vi "ReadMeanStdDevTrac.vi"(10 "error in":errorcluster, 11 "reference in 3":refnum<visa-resource-name>) -> (0 "error out 2":errorcluster, 1 "STDDEV":string, 2 "MEAN":string, 3 "TRACEr":string, 5 "reference out 4":refnum<visa-resource-name>)   [LabVIEW 2009]
panel:
  out "error out":errorcluster
  out "return count":u32
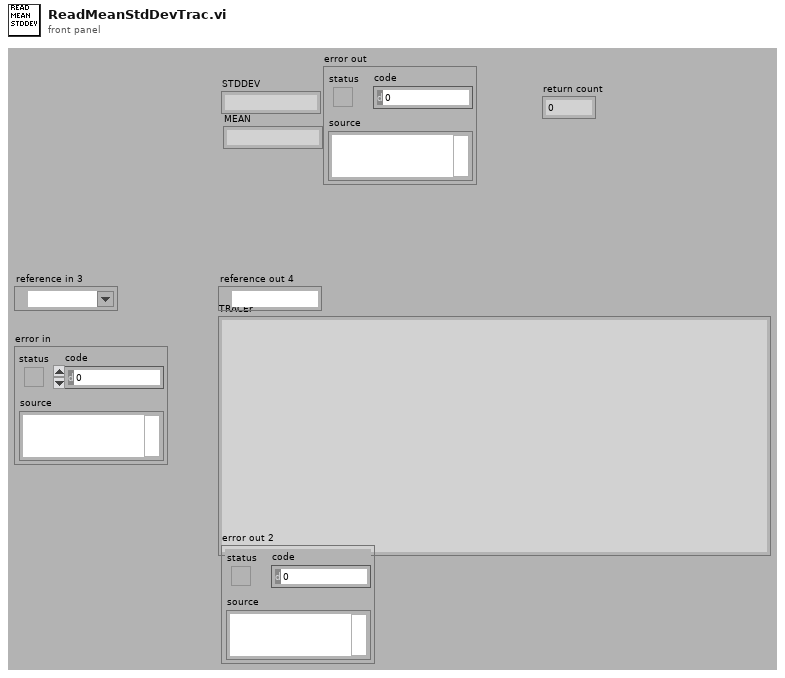
[diagram p1: front panel]
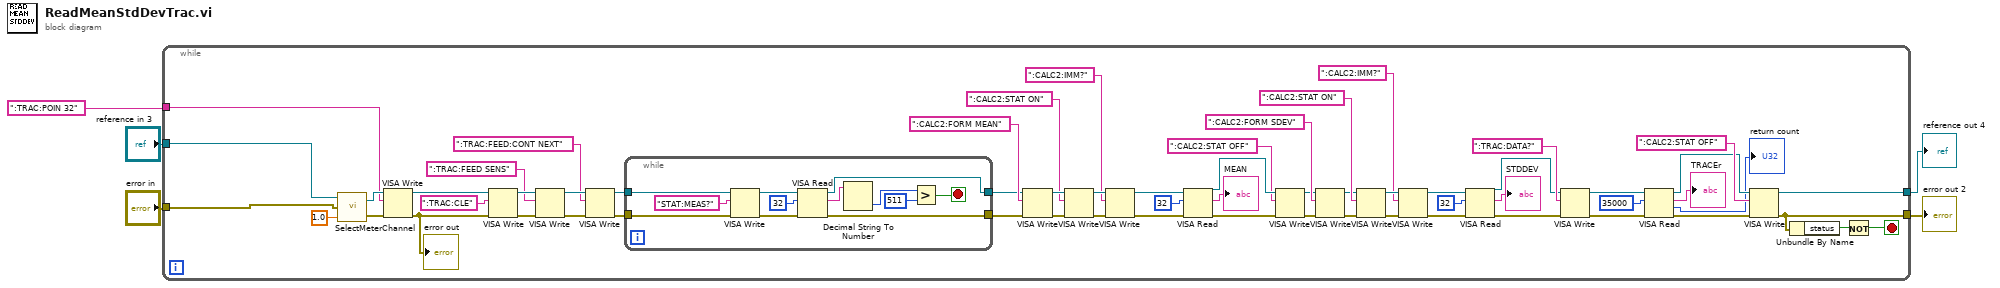
[diagram p0: block diagram]
diagram:
  n1 = while {
    tunnel: "error in" -> [w6]
    tunnel: "reference in 3" -> [w7]
    tunnel: ":TRAC:POIN 32" ("write buffer") -> [w11]
    tunnel: [w16] -> w2
    tunnel: [w28] -> w1
    stop <- w14 stop-if-true
    n2 = call "SelectMeterChannel.vi"("ChannelSelection"=1.0, "error out"=w6, "reference out"=w7) -> ("error out 2"=w13:errorcluster, "reference out 2"=w12:refnum<visa-resource-name>)
    n3 = VISA Write(VISA resource name=w12, write buffer=w11, error in (no error)=w13) -> (VISA resource name out=w8:refnum<visa-resource-name>, error out=w9:errorcluster)  [unwired: 1 out]
    "error out" <- w9
    n4 = VISA Write(VISA resource name=w8, write buffer=":TRAC:CLE", error in (no error)=w9) -> (VISA resource name out=w39:refnum<visa-resource-name>, error out=w38:errorcluster)  [unwired: 1 out]
    n5 = VISA Write(VISA resource name=w39, write buffer=":TRAC:FEED SENS", error in (no error)=w38) -> (VISA resource name out=w37:refnum<visa-resource-name>, error out=w36:errorcluster)  [unwired: 1 out]
    n6 = VISA Write(VISA resource name=w37, write buffer=":TRAC:FEED:CONT NEXT", error in (no error)=w36) -> (VISA resource name out=w34:refnum<visa-resource-name>, error out=w35:errorcluster)  [unwired: 1 out]
    n7 = while {
      tunnel: w34 -> [w78]
      tunnel: w35 -> [w77]
      tunnel: [w75] -> w19
      tunnel: [w74] -> w18
      stop <- w76 stop-if-true
      n8 = VISA Write(VISA resource name=w78, write buffer="STAT:MEAS?", error in (no error)=w77) -> (VISA resource name out=w71:refnum<visa-resource-name>, error out=w70:errorcluster)  [unwired: 1 out]
      n9 = VISA Read(VISA resource name=w71, byte count=u32 32, error in (no error)=w70) -> (VISA resource name out=w75:refnum<visa-resource-name>, read buffer=w69:string, error out=w74:errorcluster)  [unwired: 1 out]
      n10 = Decimal String To Number(string=w69) -> (number=w68:i32)  [unwired: 2 in, 1 out]
      n11 = Greater?(x=w68, y=511) -> (0:w76:bool)
    }
    n12 = VISA Write(VISA resource name=w19, write buffer=":CALC2:FORM MEAN", error in (no error)=w18) -> (VISA resource name out=w63:refnum<visa-resource-name>, error out=w62:errorcluster)  [unwired: 1 out]
    n13 = VISA Write(VISA resource name=w63, write buffer=":CALC2:STAT ON", error in (no error)=w62) -> (VISA resource name out=w60:refnum<visa-resource-name>, error out=w59:errorcluster)  [unwired: 1 out]
    n14 = VISA Write(VISA resource name=w60, write buffer=":CALC2:IMM?", error in (no error)=w59) -> (VISA resource name out=w57:refnum<visa-resource-name>, error out=w56:errorcluster)  [unwired: 1 out]
    n15 = VISA Read(VISA resource name=w57, byte count=u32 32, error in (no error)=w56) -> (VISA resource name out=w25:refnum<visa-resource-name>, read buffer=→"MEAN":string, error out=w26:errorcluster)  [unwired: 1 out]
    n16 = VISA Write(VISA resource name=w25, write buffer=":CALC2:STAT OFF", error in (no error)=w26) -> (VISA resource name out=w24:refnum<visa-resource-name>, error out=w23:errorcluster)  [unwired: 1 out]
    n17 = VISA Write(VISA resource name=w24, write buffer=":CALC2:FORM SDEV", error in (no error)=w23) -> (VISA resource name out=w21:refnum<visa-resource-name>, error out=w20:errorcluster)  [unwired: 1 out]
    n18 = VISA Write(VISA resource name=w21, write buffer=":CALC2:STAT ON", error in (no error)=w20) -> (VISA resource name out=w53:refnum<visa-resource-name>, error out=w52:errorcluster)  [unwired: 1 out]
    n19 = VISA Write(VISA resource name=w53, write buffer=":CALC2:IMM?", error in (no error)=w52) -> (VISA resource name out=w44:refnum<visa-resource-name>, error out=w45:errorcluster)  [unwired: 1 out]
    n20 = VISA Read(VISA resource name=w44, byte count=u32 32, error in (no error)=w45) -> (VISA resource name out=w43:refnum<visa-resource-name>, read buffer=→"STDDEV":string, error out=w42:errorcluster)  [unwired: 1 out]
    n21 = VISA Write(VISA resource name=w43, write buffer=":TRAC:DATA?", error in (no error)=w42) -> (VISA resource name out=w48:refnum<visa-resource-name>, error out=w47:errorcluster)  [unwired: 1 out]
    n22 = VISA Read(VISA resource name=w48, byte count=u32 35000, error in (no error)=w47) -> (VISA resource name out=w30:refnum<visa-resource-name>, read buffer=→"TRACEr":string, return count=→"return count":u32, error out=w29:errorcluster)
    n23 = VISA Write(VISA resource name=w30, write buffer=":CALC2:STAT OFF", error in (no error)=w29) -> (VISA resource name out=w28:refnum<visa-resource-name>, error out=w16:errorcluster)  [unwired: 1 out]
    n24 = Unbundle By Name(w16) -> ("status"=w15:bool)
    n25 = Not(x=w15) -> (.not. x?=w14:bool)
  }
  "error out 2" <- w2
  "reference out 4" <- w1
